vi "fpga_integrator_AOD_random_access_motion.vi"(8 "error in":errorcluster) -> (0 "error out":errorcluster)   [LabVIEW 2010]
uses:
  fpgaVIsAndControls/DDS_board_init_cluster.ctl
  fpgaVIsAndControls/FPGA_parameters_cluster.ctl
  common_typedefs/channels_cluster.ctl
  fpgaVIsAndControls/scan_points_cluster.ctl
  fpgaVIsAndControls/ellipsoid_parameters_cluster.ctl
  fpgaVIsAndControls/anti-photo-bleaching_rotation_cluster.ctl
  common_typedefs/gate_parameters_cluster.ctl
  <vilib>/Platform/TimedLoop/XDataNode/XDataNode.xnode
  <vilib>/Platform/TimedLoop/XDataNode/timing_clust.ctl
  <vilib>/Platform/TimedLoop/XDataNode/nitl_modes.ctl
  <vilib>/Platform/TimedLoop/XDataNode/wakeup.ctl
  <vilib>/eio/EIONode/EIONode.xnode
  <vilib>/rvi/eio/nirviEIOImplementation/nirviEIOImplementation.xnode
  <vilib>/rvi/eio/common/nirviEmuClasses.ctl
  <vilib>/rvi/eio/nirviErrorMerge/nirviErrorMerge.xnode
  <vilib>/rvi/DataTransferAndStorage/Container/XNode/niFpgaContainer.xnode
  <vilib>/rvi/eio/common/nirviEmuTemplateMethod_errors.vi
  <vilib>/rvi/eio/common/nirviEmuTemplateMethod_noerrors.vi
  <vilib>/rvi/FIFO/Fifo_Resource/nirvififoEmulationSetSize.vi
  <vilib>/rvi/DataTransferAndStorage/Container/Common/niFpgaContainerGetUniqueNameForEmu.vi
  <vilib>/Platform/TimedLoop/XDataNode/XDNodeRunTimeDep.lvlib
panel:
  in  "integration delay (iterations)":i32
  in  "integration delay (pixels)":i32
  in  "first pixel black?":bool
  in  "gate 1":T1
  in  "gate 2":T1
  in  "gate 3":T1
  out "clock 2 state":bool
  out "clock 1 state":bool
  out "clock 3 state":bool
  out "acquiring?":bool
  in  "sub-pattern iterations per pixel":u16
  out "rotation cluster out":T2={"ellipsoid"={"counter"=0, "~x n"=0.999969482421875, "~y n"=0.0, "~z n"=5.0, "amp 0"=0.0}} {"ellipsoid"."amp 0" format="%.16g"; "ellipsoid"."~y n" format="%.16g"; "ellipsoid"."~x n" format="%.16g"}
  in  "ellipsoid parameter cluster":T3={"a"=0.0, "b"=0.125, "c"=0.5, "d"=0.015625, "e"=0.5, "k"=50, "width"=0.0} {"a" format="%.16g"; "b" format="%.16g"; "c" format="%.16g"; "d" format="%.16g"}
  in  "in triggered mode?":bool
  in  "stop at FIFO overflow?":bool
  in  "converter box version":i16=1 min=1 max=2
  out "counter in":i32
  out "reset out":bool
  out "scan points cluster out":T4
  in  "ra trajectory pixels\n(data/pixels transfered)":u32=65535
  out "FIFO scan time out":bool
  in  "y-point bandwidth":fxp<+,36,32>=10.0 format="%.28g"
  in  "x-point bandwidth":fxp<+,36,32>=10.0 format="%.28g"
  in  "amp comp":bool
  in  "inverse?":T5(ring)
  in  "OSK select":bool=TRUE
  in  "FPGA parameters in":T6 {"AOD center frequ. (Hz)_y" format="%.14g"; "AOD half bandwidth_y" format="%.14g"; "AOD Bandwidth_y (Hz)" format="%_6f"; "AOD center frequ. (Hz)_x" format="%.14g"; "cos Phi" format="%.35g"; "sin Phi" format="%.35g"; "AOD_Scale_Factor (1/Zoom)" format="%.35g"; "AOD half bandwidth_x" format="%.14g"; "AOD Bandwidth_x (Hz)" format="%_6f"}
  out "integrated pixel values":T7
  in  "maximum bit depth":i8=16
  in  "intergration iterations per pixel":u32=40
  in  "waiting iterations  per pixel":u32=200
  out "data read":T7
  in  "channel offsets":T7
  in  "number of pixels":i64=-1
  out "FIFO_DMA0 full?":bool
  out "current pixel no.":i64
  out "FPGA parameters out":T6 {"AOD center frequ. (Hz)_y" format="%.14g"; "AOD half bandwidth_y" format="%.14g"; "AOD Bandwidth_y (Hz)" format="%_6f"; "AOD center frequ. (Hz)_x" format="%.14g"; "cos Phi" format="%.35g"; "sin Phi" format="%.35g"; "AOD_Scale_Factor (1/Zoom)" format="%.35g"; "AOD half bandwidth_x" format="%.14g"; "AOD Bandwidth_x (Hz)" format="%_6f"}
  in  "acquire?":bool caption="Acquire?"
  in  "Stop complete VI":bool caption="Stop"
  in  "reset in":bool caption="Reset"
  in  "DDS board initialization parameters":T8={"Bypass PLL"=FALSE, "PLL Range"=TRUE, "Update Clock"=FALSE, "Triangle "=FALSE, "SDO Active"=FALSE, "LSB First"=FALSE, "OSK Int"=FALSE, "Output Shaped Keying Enable"=TRUE, "Bypass Sinc"=FALSE, "Digital Part"=TRUE, "OutPut DAC"=TRUE, "Control DAC"=TRUE, "Comparator"=FALSE, "Modus"=0, "Multiplier Value"=15} {"Modus" scale=0.0..4.0}
  # "FPGA integrator"
  # "IN"
  # "OUT"
  # "DDS"
  # "Clock parameters"
  # "DIO 1/32"
  # "PXI/RTSI 1"
  # "PXI/RTSI 2"
  # "FSK"
  # "Ramped"
  # "FSK"
  # "Chirp Modus"
  # "Unramped"
  # "BPSK"
  # "Single Tone"
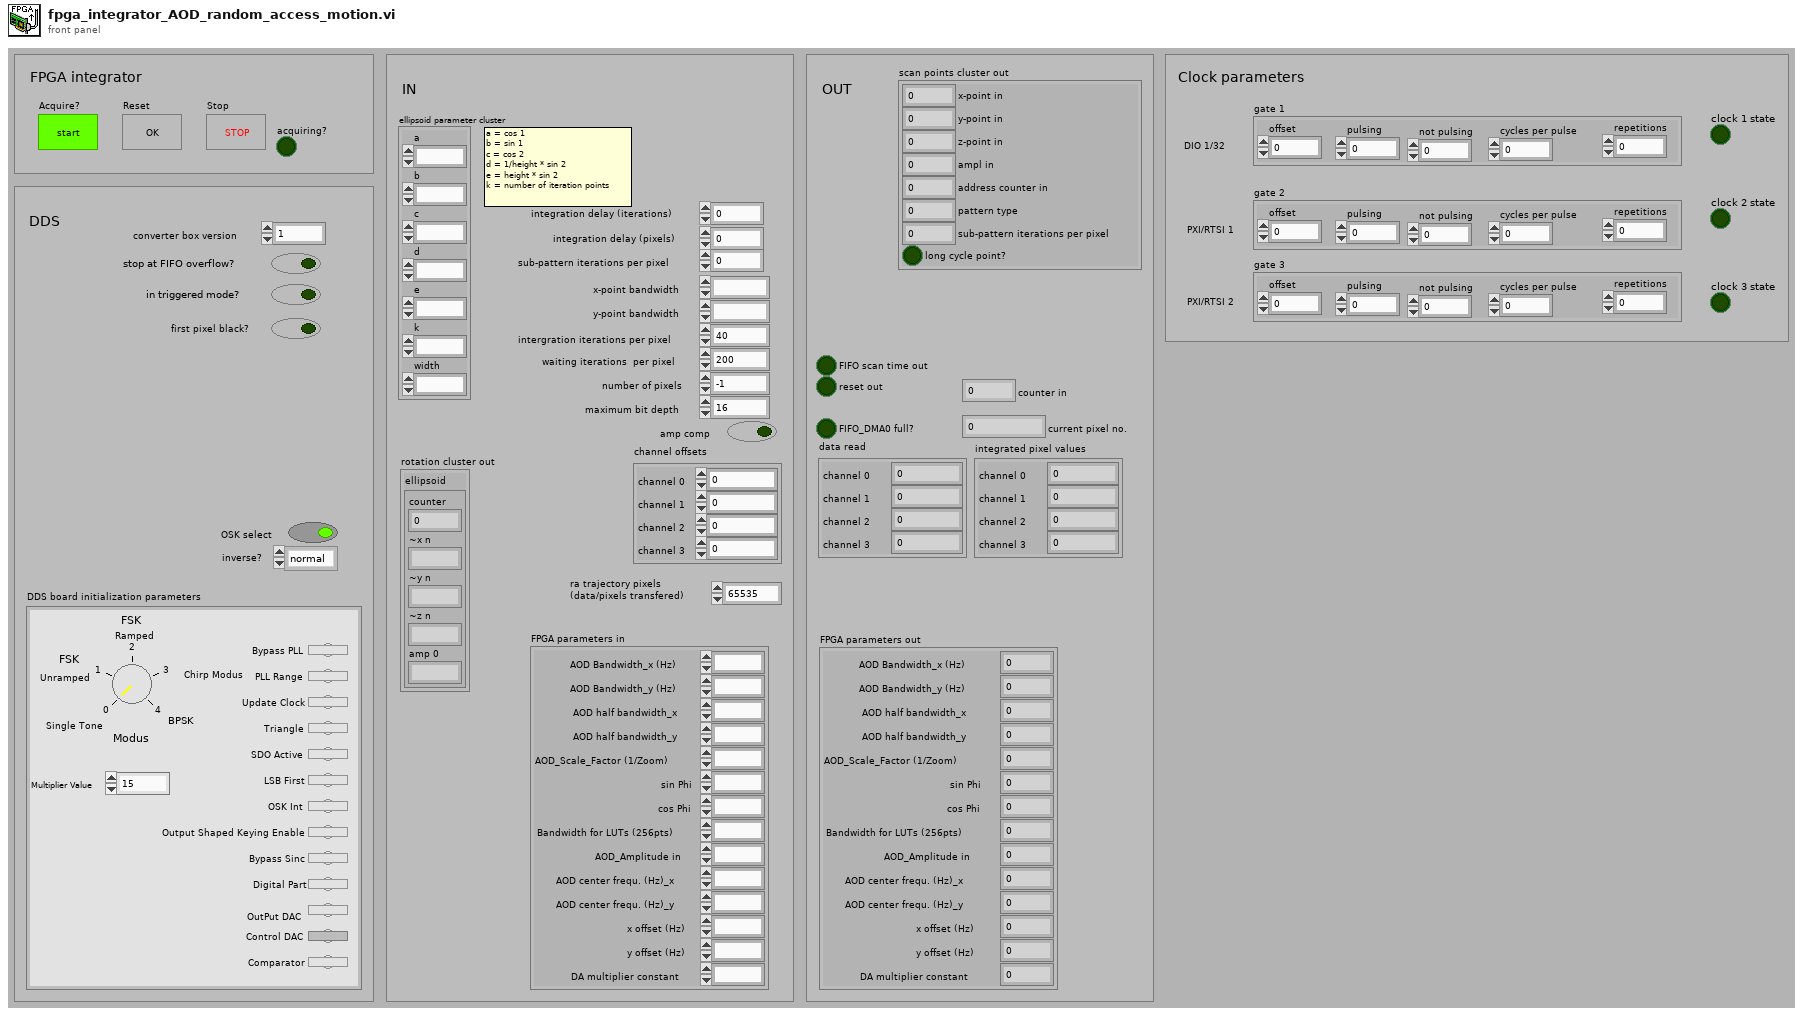
[diagram p1: front panel]
types:
  T1 = typedef "gate_parameters_cluster.ctl" = cluster{"offset":i64, "pulsing":i64, "not pulsing":i64, "cycles per pulse":i64, "repetitions":i64}
  T2 = typedef "anti-photo-bleaching_rotation_cluster.ctl" = cluster{"ellipsoid":cluster{"counter":u16, "~x n":fxp<+/-,16,1>, "~y n":fxp<+/-,16,1>, "~z n":fxp<+/-,32,16>, "amp 0":fxp<+/-,16,1>}}
  T3 = typedef "ellipsoid_parameters_cluster.ctl" = cluster{"a":fxp<+/-,16,1>, "b":fxp<+/-,16,1>, "c":fxp<+/-,16,1>, "d":fxp<+/-,16,1>, "e":fxp<+/-,24,16>, "k":u16, "width":fxp<+,16,16>}
  T4 = typedef "scan_points_cluster.ctl" = cluster{"x-point in":i32, "y-point in":i32, "z-point in":i32, "ampl in":u16, "address counter in":i32, "pattern type":i8, "sub-pattern iterations per pixel":u16, "long cycle point?":bool}
  T5 = enum16{"normal", "x inversed", "y inversed", "x & y inversed"}
  T6 = typedef "FPGA_parameters_cluster.ctl" = cluster{"AOD Bandwidth_x (Hz)":fxp<+,36,32>, "AOD Bandwidth_y (Hz)":fxp<+,36,32>, "AOD half bandwidth_x":fxp<+,36,32>, "AOD half bandwidth_y":fxp<+,36,32>, "AOD_Scale_Factor (1/Zoom)":fxp<+,36,2>, "sin Phi":fxp<+/-,36,2>, "cos Phi":fxp<+/-,36,2>, "Bandwidth for LUTs (256pts)":fxp<+,36,0>, "AOD_Amplitude in":u16, "AOD center frequ. (Hz)_x":fxp<+,36,32>, "AOD center frequ. (Hz)_y":fxp<+,36,32>, "x offset (Hz)":fxp<+/-,36,32>, "y offset (Hz)":fxp<+/-,36,32>, "DA multiplier constant":fxp<+,64,4>}
  T7 = typedef "channels_cluster.ctl" = cluster{"channel 0":u32, "channel 1":u32, "channel 2":u32, "channel 3":u32}
  T8 = typedef "DDS_board_init_cluster.ctl" = cluster{"Bypass PLL":bool, "PLL Range":bool, "Update Clock":bool, "Triangle ":bool, "SDO Active":bool, "LSB First":bool, "OSK Int":bool, "Output Shaped Keying Enable":bool, "Bypass Sinc":bool, "Digital Part":bool, "OutPut DAC":bool, "Control DAC":bool, "Comparator":bool, "Modus":u8, "Multiplier Value":u8}
  T9 = typedef "FPGA_constants_cluster.ctl" = cluster{"register":cluster{"Reg. 1D":u8, "Reg. 1E":u8, "Reg. 1F":u8, "Reg. 20":u8}}
  T10 = typedef "XDNodeRunTimeDep.lvlib/timing_clust.ctl" = cluster{"Expected End [f-1]":u64, "Actual End [f-1]":u64, "Finished Late? [f-1]":bool, "Expected End [i-1]":u64, "Actual End [i-1]":u64, "Finished Late? [i-1]":bool, "Expected Start [i]":u64, "Actual Start [i]":u64, "Expected Start [f]":u64, "Actual Start [f]":u64, "Source Name":string, "Structure Name":string, "Period":i64, "Deadline":i64, "Offset":i64, "Start":i64, "Priority":i32, "Timeout":i32, "Mode":T11, "Wakeup Reason":T12, "Error":errorcluster, "Source Type":string, "Secondary Source Type":string, "Global End Time":u64, "Global Start Time":u64, "Frame Duration":u64, "Iteration Duration":u64, "Assigned CPU":i32, "I/O Scan Engine Mode":u32}
  T11 = typedef "XDNodeRunTimeDep.lvlib/nitl_modes.ctl" = enum32{"No Change", "Process missed periods, maintain original phase", "Discard missed periods, maintain original phase", "Process missed periods, ignore original phase", "Discard missed periods, ignore original phase"}
  T12 = typedef "XDNodeRunTimeDep.lvlib/wakeup.ctl" = enum32{"Normal", "Aborted", "Asynchronous wakeup", "Timing source error", "Timed loop error", "Timeout"}
  T13 = typedef "DDS_board_values_cluster.ctl" = cluster{"y-frequency output":fxp<+,36,32>, "y-amplitude output":u16, "x-amplitude output":u16, "x-frequency output":fxp<+,36,32>, "z-position output":i16}
  T14 = typedef "nirviEmuClasses.ctl" = enum16{"IO Read", "IO Write", "Method", "Property Read", "Property Write"}
  T15 = typedef "gate_counters_cluster.ctl" = cluster{"phase iteration counter":i64, "phase repetition counter":i64, "pulse iteration counter":i64, "phase state":bool}
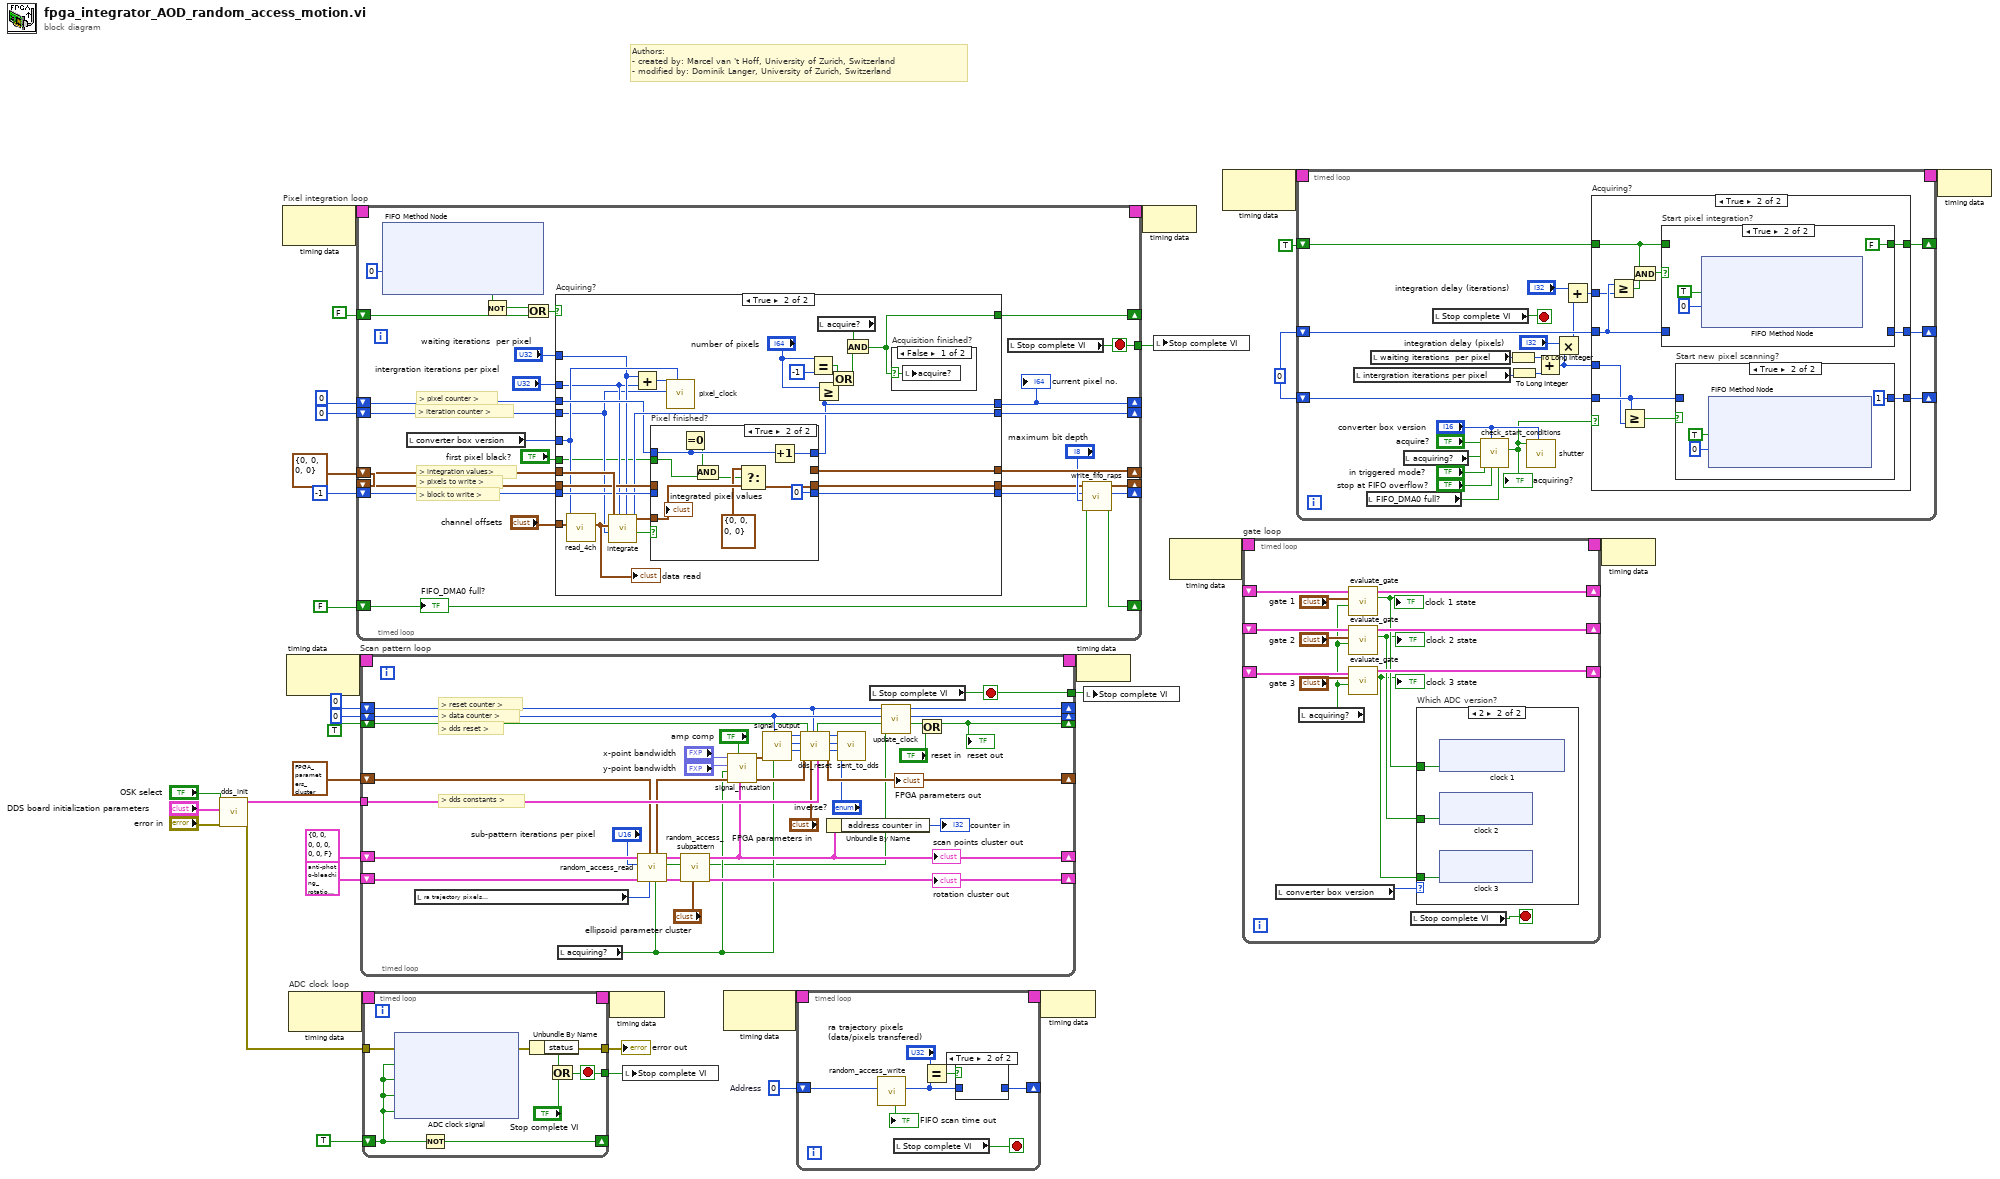
[diagram p0: block diagram]
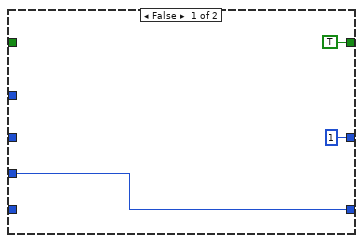
[diagram p2: hidden frame]
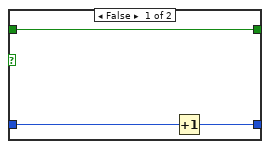
[diagram p3: hidden frame]
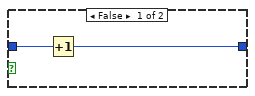
[diagram p4: hidden frame]
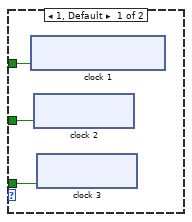
[diagram p5: hidden frame]
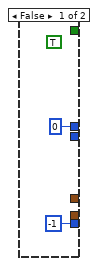
[diagram p7: hidden frame]
diagram:
  w3 = 0
  w10 = u32 0  # Address
  w19 = T7 {"channel 0"=0, "channel 1"=0, "channel 2"=0, "channel 3"=0} ("channel offsets 2")
  # "Authors: \n- created by: Marcel van 't Hoff, University of Zurich, Switzerland\n- modified by: Dominik Langer, University of Zurich, Switzerland"
  n1 = call "dds_init.vi"("error in"="error in", "DDS board initialization parameters"="DDS board initialization parameters", "OSK select"="OSK select") -> ("error out"=w31:errorcluster, "constants out"=w32:T9)  [unwired: 7 in]
  n2 = node-c288() -> (w27:T10)  [unwired: 1 out]
  n3 = node-c288() -> (w21:T10)  [unwired: 1 in]
  n4 = node-c288() -> (w37:T10)  [unwired: 1 out]
  n5 = timed-loop "Pixel integration loop" {
    timing: w27 -> [_]
    timing-out: [_] -> w26
    shift-right: [w64] -> _
    shift-left: w19 -> [w63]
    shift-right: [w49] -> _
    shift-left: w19 -> [w62]
    shift-right: [w46] -> _
    shift-left: -1 ("block index out") -> [w61]
    shift-right: [w59] -> _
    shift-left: u32 0 ("iteration counter out") -> [w60]
    shift-right: [w57] -> _
    shift-left: i64 0 -> [w58]
    tunnel: [w56] -> w22
    shift-right: [w50] -> _
    shift-left: FALSE -> [w51]
    shift-right: [w39] -> _
    shift-left: FALSE -> [w41]
    stop <- w56 stop-if-true
    # "> pixel counter >"
    # "> block to write >"
    # "> integration values>"
    # "> pixels to write >"
    # "> iteration counter >"
    n6 = xnode ("FIFO Method Node")("Timeout"=0) -> ("Timed Out?"=w44:bool)  [unwired: 1 in, 2 out]
    n7 = local read "converter box version"() -> (w45:i16)
    n8 = Not(x=w44) -> (.not. x?=w42:bool)
    n9 = Or(x=w42, y=w41) -> (x .or. y?=w40:bool)
    n10 = case "Acquiring?" shown="True" w40 {
      tunnel: [_ w140] -> w64
      tunnel: w63 -> [_ w143]
      tunnel: [_ w125] -> w48
      tunnel: w62 -> [_ w138]
      tunnel: [-1 ("block index out") w126] -> w47
      tunnel: w61 -> [_ w139]
      tunnel: w60 -> [_ w121]
      tunnel: [_ w137] -> w59
      tunnel: w58 -> [_ w129]
      tunnel: [i64 0 w128] -> w57
      tunnel: "channel offsets" -> [_ w127]
      tunnel: "intergration iterations per pixel" -> [_ w122]
      tunnel: "waiting iterations  per pixel" -> [_ w123]
      tunnel: w45 -> [_ w124]
      tunnel: [_ w119] -> w39
      tunnel: "first pixel black?" -> [_ w118]
      frame False {
        (unwired) TRUE
      }
      frame True {
        n11 = call "read_4ch.vi"("channel offsets"=w127, "converter box version"=w124) -> ("read output"=w141:T7)  [unwired: 9 in]
        "data read" <- w141
        n12 = call "integrate.vi"("waiting iterations per pixel"=w123, "integration iterations per pixel"=w122, "iteration counter in"=w121, "sampling values in"=w141, "previous pixel values in"=w143) -> ("finished?"=w131:bool, "iteration counter out"=w137:u32, "new pixel values out"=w142:T7)  [unwired: 4 in]
        n13 = Add(x=w123, y=w122) -> (x+y=w120:u32)
        n14 = case "Pixel finished?" shown="True" w131 {
          tunnel: w142 -> [w148 w154]
          tunnel: [w148 _] -> w140
          tunnel: w139 -> [w147 _]
          tunnel: [w147 0 ("block index out")] -> w126
          tunnel: w138 -> [w146 _]
          tunnel: [w146 w153] -> w125
          tunnel: w129 -> [w145 w155]
          tunnel: [w145 w157] -> w128
          tunnel: w118 -> [_ w150]
          frame False {
          }
          frame True {
            n15 = Equal To 0?(x=w155) -> (x = 0?=w151:bool)
            n16 = And(x=w151, y=w150) -> (x .and. y?=w149:bool)
            n17 = Select(t=T7 {"channel 0"=0, "channel 1"=0, "channel 2"=0, "channel 3"=0}, s=w149, f=w154) -> (s? t:f=w153:T7)
            n18 = Increment(x=w155) -> (x+1=w157:i64)
            "integrated pixel values" <- w154
          }
        }
        n19 = call "pixel_clock.vi"("converter box version"=w124, "current iteration"=w121, "iterations per pixel"=w120) -> ()  [unwired: 9 in]
        n20 = Equal?(x="number of pixels", y=i64 -1 ("x")) -> (x = y?=w134:bool)
        n21 = Greater Or Equal?(x="number of pixels", y=w128) -> (x >= y?=w133:bool)
        n22 = local read "acquire?"() -> (w136:bool)
        n23 = Or(x=w134, y=w133) -> (x .or. y?=w135:bool)
        n24 = And(x=w136, y=w135) -> (x .and. y?=w119:bool)
        n25 = case "Acquisition finished?" shown="False" w119 {
          selector: w119 -> [w144 _]
          frame False {
            n26 = local write "acquire?"(w144) -> ()
          }
          frame True {
          }
        }
      }
    }
    "current pixel no." <- w57
    n27 = local read "Stop complete VI"() -> (w56:bool)
    n28 = call "write_fifo_raps.vi"("FIFO overflow in"=w51, "maximum bit depth"="maximum bit depth", "block index in"=w47, "values to be written"=w48) -> ("FIFO overflow out"=w50:bool, "block index out"=w46:i32, "channels out"=w49:T7)  [unwired: 5 in]
    "FIFO_DMA0 full?" <- w51
  }
  n29 = timed-loop "Scan pattern loop" {
    tunnel: [w174] -> w33
    tunnel: w32 -> [w186]
    shift-right: [w183] -> _
    shift-left: T6 {"AOD Bandwidth_x (Hz)"=35000000.0, "AOD Bandwidth_y (Hz)"=35000000.0, "AOD half bandwidth_x"=17500000.0, "AOD half bandwidth_y"=17500000.0, "AOD_Scale_Factor (1/Zoom)"=0.0, "sin Phi"=0.0, "cos Phi"=1.0, "Bandwidth for LUTs (256pts)"=0.0, "AOD_Amplitude in"=1, "AOD center frequ. (Hz)_x"=0.0, "AOD center frequ. (Hz)_y"=3400.0, "x offset (Hz)"=94000000.0, "y offset (Hz)"=94000000.0, "DA multiplier constant"=0.0} ("FPGA parameters out 2") -> [w176]
    shift-right: [w193] -> _
    shift-left: TRUE ("reset dds out") -> [w173]
    shift-right: [w191] -> _
    shift-left: u32 0 ("data sending counter (#bytes) out") -> [w190]
    shift-right: [w189] -> _
    shift-left: u8 0 ("reset counter out") -> [w185]
    timing: w21 -> [_]
    timing-out: [_] -> w20
    shift-right: [w169] -> _
    shift-left: T4 {"x-point in"=0, "y-point in"=0, "z-point in"=0, "ampl in"=0, "address counter in"=0, "pattern type"=0, "sub-pattern iterations per pixel"=0, "long cycle point?"=FALSE} ("scan points cluster out") -> [w167]
    shift-right: [w171] -> _
    shift-left: T2 {"ellipsoid"={"counter"=0, "~x n"=0.999969482421875, "~y n"=0.0, "~z n"=5.0, "amp 0"=0.0}} ("rotation cluster out") -> [w165]
    stop <- w174 stop-if-true
    # "> dds constants >"
    # "> dds reset >"
    # "> data counter >"
    # "> reset counter >"
    n30 = local read "ra trajectory pixels\n(data/pixels transfered)"() -> (w168:u32)
    n31 = local read "acquiring?"() -> (w162:bool)
    n32 = call "random_access_read.vi"("ra scanning?"=w162, "ra trajectory pixels (data/pixels transfered)"=w168, "FPGA parameters in"=w176, "rotation cluster in"=w165, "sub-pattern iterations per pixel"="sub-pattern iterations per pixel", "scan points cluster in"=w167) -> ("rotation cluster out"=w164:T2, "new pixel update?"=w161:bool, "scan points cluster out"=w166:T4, "FPGA parameters out"=w175:T6)  [unwired: 2 in]
    n33 = call "random_access_subpattern.vi"("ellipsoid parameter cluster"="ellipsoid parameter cluster", "rotation cluster in"=w164, "new pixel? in"=w161, "scan points cluster in"=w166) -> ("rotation cluster out"=w171:T2, "next pixel? out"=w160:bool, "scan points cluster out"=w169:T4)  [unwired: 5 in]
    "scan points cluster out" <- w169
    "rotation cluster out" <- w171
    n34 = call "signal_mutation.vi"("scan points cluster in"=w169, "amplitude compensation?"="amp comp", "FPGA parameters in"=w175, "acquire?"=w162, "y point bandwidth"="y-point bandwidth", "x point bandwidth"="x-point bandwidth") -> ("FPGA parameters out"=w180:T6, "cluster out"=w192:T13)  [unwired: 4 in]
    n35 = call "signal_output.vi"("acquire?"=w162, "pipeline counter in"=w190, "cluster in"=w192) -> ("address bits out"=w197:u8, "y data bits out"=w198:u8, "x data bits out"=w199:u8)  [unwired: 6 in]
    n36 = call "dds_reset.vi"("DDS data bits in"=w199, "DDS0 data bits in"=w198, "address bits in"=w197, "FPGA parameters in"=w180, "reset dds in"=w173, "counter in"=w185, "FPGA parameters reset"="FPGA parameters in", "constants in"=w186) -> ("reset dds out"=w188:bool, "DDS0 data bits out"=w196:u8, "DDS1 data bits out"=w195:u8, "address bits out"=w194:u8, "FPGA parameters out"=w183:T6)  [unwired: 7 in]
    "FPGA parameters out" <- w183
    n37 = Unbundle By Name(w169) -> ("address counter in"=→"counter in":i32)
    n38 = call "sent_to_dds.vi"("inversion selector"="inverse?", "address bits in"=w194, "DDS1 input"=w195, "DDS0 input"=w196) -> ()  [unwired: 8 in]
    n39 = local read "Stop complete VI"() -> (w174:bool)
    n40 = call "update_clock.vi"("update command in"=w160, "update reset counter in"=w188, "data sending counter (#bytes) in"=w190, "reset counter in"=w185) -> ("update reset counter out"=w184:bool, "data sending counter (#bytes) out"=w191:u32, "reset counter out"=w189:u8)  [unwired: 5 in]
    n41 = Or(x=w184, y="reset in") -> (x .or. y?=w193:bool)
    "reset out" <- w193
  }
  n42 = timed-loop "ADC clock loop" {
    timing: w37 -> [_]
    timing-out: [_] -> w36
    shift-right: [w203] -> _
    shift-left: TRUE -> [w208]
    tunnel: [w205] -> w34
    tunnel: w31 -> [w204]
    tunnel: [w202] -> w18
    stop <- w205 stop-if-true
    n43 = xnode "ADC clock signal"("error in"=w204, "Connector0/DIO14"=w208, "Connector0/DIO15"=w208, "Connector1/DIO14"=w208, "Connector1/DIO15"=w208) -> ("error out"=w202:errorcluster)  [unwired: 4 in, 4 out]
    n44 = Not(x=w208) -> (.not. x?=w203:bool)
    n45 = Unbundle By Name(w202) -> ("status"=w206:bool)
    n46 = Or(x=w206, y="Stop complete VI") -> (x .or. y?=w205:bool)
  }
  "error out" <- w18
  n47 = node-c288(w36) -> ()
  n48 = local write "Stop complete VI"(w34) -> ()
  n49 = node-c288() -> (w12:T10)  [unwired: 1 in]
  n50 = timed-loop {
    timing: w12 -> [_]
    timing-out: [_] -> w11
    shift-right: [w307] -> _
    shift-left: w10 -> [w308]
    stop <- w306 stop-if-true
    n51 = call "random_access_write.vi"("address in"=w308) -> ("address out"=w310:u32, "FIFO scan time out"=→"FIFO scan time out":bool)  [unwired: 9 in]
    n52 = local read "Stop complete VI"() -> (w306:bool)
    n53 = Equal?(x="ra trajectory pixels\n(data/pixels transfered)", y=w310) -> (x = y?=w311:bool)
    n54 = case shown="True" w311 {
      tunnel: [w313 _] -> w307
      tunnel: w310 -> [w313 _]
      frame False {
      }
      frame True {
      }
    }
  }
  n55 = node-c288(w11) -> ()
  n56 = node-c288(w20) -> ()
  n57 = local write "Stop complete VI"(w33) -> ()
  n58 = node-c288(w26) -> ()
  n59 = local write "Stop complete VI"(w22) -> ()
  n60 = node-c288() -> (w8:T10)  [unwired: 1 in]
  n61 = node-c288() -> (w5:T10)  [unwired: 1 in]
  n62 = timed-loop "gate loop" {
    timing: w8 -> [_]
    timing-out: [_] -> w7
    shift-right: [w329] -> _
    shift-left: _ -> [w330]
    shift-right: [w327] -> _
    shift-left: _ -> [w328]
    shift-right: [w326] -> _
    shift-left: _ -> [w325]
    stop <- w317 stop-if-true
    n63 = local read "converter box version"() -> (w318:i16)
    n64 = local read "acquiring?"() -> (w316:bool)
    n65 = call "evaluate_gate.vi"("acquiring?"=w316, "gate settings"="gate 1", "gate counters in"=w330) -> ("pulse state out"=w321:bool, "gate counters out"=w329:T15)  [unwired: 7 in]
    "clock 1 state" <- w321
    n66 = call "evaluate_gate.vi"("acquiring?"=w316, "gate settings"="gate 2", "gate counters in"=w328) -> ("pulse state out"=w320:bool, "gate counters out"=w327:T15)  [unwired: 7 in]
    "clock 2 state" <- w320
    n67 = call "evaluate_gate.vi"("acquiring?"=w316, "gate settings"="gate 3", "gate counters in"=w325) -> ("pulse state out"=w319:bool, "gate counters out"=w326:T15)  [unwired: 7 in]
    "clock 3 state" <- w319
    n68 = local read "Stop complete VI"() -> (w317:bool)
    n69 = case "Which ADC version?" shown="2" w318 {
      tunnel: w321 -> [w331 w369]
      tunnel: w320 -> [w332 w368]
      tunnel: w319 -> [w333 w367]
      frame 1, Default {
        n70 = xnode "clock 1"("Connector1/DIO32"=w331) -> ()  [unwired: 1 in, 1 out]
        n71 = xnode "clock 2"("PXI_RTSI_1"=w332) -> ()  [unwired: 1 in, 1 out]
        n72 = xnode "clock 3"("PXI_RTSI_2"=w333) -> ()  [unwired: 1 in, 1 out]
      }
      frame 2 {
        n73 = xnode "clock 1"("Connector0/DIO38"=w369) -> ()  [unwired: 1 in, 1 out]
        n74 = xnode "clock 2"("PXI_RTSI_1"=w368) -> ()  [unwired: 1 in, 1 out]
        n75 = xnode "clock 3"("PXI_RTSI_2"=w367) -> ()  [unwired: 1 in, 1 out]
      }
    }
  }
  n76 = timed-loop {
    timing: w5 -> [_]
    timing-out: [_] -> w4
    shift-right: [w425] -> _
    shift-left: w3 -> [w426]
    shift-right: [w423] -> _
    shift-left: w3 -> [w424]
    shift-right: [w410] -> _
    shift-left: TRUE -> [w411]
    stop <- w427 stop-if-true
    n77 = local read "intergration iterations per pixel"() -> (w415:u32)
    n78 = local read "FIFO_DMA0 full?"() -> (w422:bool)
    n79 = local read "waiting iterations  per pixel"() -> (w414:u32)
    n80 = local read "acquiring?"() -> (w416:bool)
    n81 = local read "Stop complete VI"() -> (w427:bool)
    n82 = call "check_start_conditions.vi"("FIFO overflow?"=w422, "stop at FIFO overflow?"="stop at FIFO overflow?", "converter box version"="converter box version", "already acquiring?"=w416, "in triggered mode?"="in triggered mode?", "acquire"="acquire?") -> ("acquire?"=w418:bool)  [unwired: 5 in]
    "acquiring?" <- w418
    n83 = To Long Integer(number=w414) -> (32bit integer=w413:i32)
    n84 = To Long Integer(number=w415) -> (32bit integer=w412:i32)
    n85 = call "shutter.vi"("converter box version"="converter box version", "open?"=w418) -> ()  [unwired: 10 in]
    n86 = Add(x=w413, y=w412) -> (x+y=w409:i32)
    n87 = Multiply(x="integration delay (pixels)", y=w409) -> (x*y=w406:i32)
    n88 = Add(x="integration delay (iterations)", y=w406) -> (x+y=w405:i32)
    n89 = case "Acquiring?" shown="True" w418 {
      tunnel: w426 -> [_ w438]
      tunnel: [w430 w440] -> w425
      tunnel: w424 -> [_ w435]
      tunnel: [1 w439] -> w423
      tunnel: w409 -> [w430 w437]
      tunnel: w411 -> [_ w431]
      tunnel: [TRUE w436] -> w410
      tunnel: w405 -> [_ w434]
      frame False {
      }
      frame True {
        n90 = Greater Or Equal?(x=w435, y=w434) -> (x >= y?=w433:bool)
        n91 = Greater Or Equal?(x=w438, y=w437) -> (x >= y?=w441:bool)
        n92 = And(x=w431, y=w433) -> (x .and. y?=w432:bool)
        n93 = case "Start pixel integration?" shown="True" w432 {
          tunnel: w435 -> [w444 _]
          tunnel: [w443 _] -> w439
          tunnel: w431 -> [w442 _]
          tunnel: [w442 FALSE] -> w436
          frame False {
            n94 = Increment(x=w444) -> (x+1=w443:i32)
          }
          frame True {
            n95 = xnode ("FIFO Method Node")("Element"=TRUE, "Timeout"=0) -> ()  [unwired: 1 in, 2 out]
          }
        }
        n96 = case "Start new pixel scanning?" shown="True" w441 {
          tunnel: w438 -> [w500 _]
          tunnel: [w499 1] -> w440
          frame False {
            n97 = Increment(x=w500) -> (x+1=w499:i32)
          }
          frame True {
            n98 = xnode ("FIFO Method Node")("Element"=TRUE, "Timeout"=0) -> ()  [unwired: 1 in, 2 out]
          }
        }
      }
    }
  }
  n99 = node-c288(w7) -> ()
  n100 = node-c288(w4) -> ()
